vi "Qn10_X.vi"(11 "String":string) -> (3 "Qn":dbl[](array[numeric]))   [LabVIEW 2015]
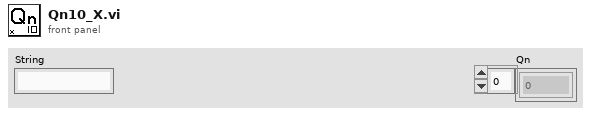
[diagram p1: front panel]
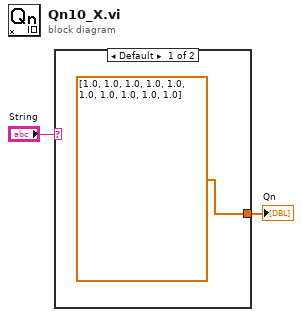
[diagram p0: block diagram]
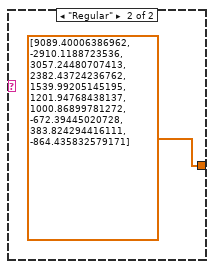
[diagram p2: hidden frame]
diagram:
  n1 = case shown="Default" "String" {
    tunnel: [dbl[] [1.0, 1.0, 1.0, 1.0, 1.0, 1.0, 1.0, 1.0, 1.0, 1.0] ("Qn") dbl[] [9089.40006386962, -2910.1188723536, 3057.24480707413, 2382.43724236762, 1539.99205145195, 1201.94768438137, 1000.86899781272, -672.39445020728, 383.824294416111, -864.435832579171] ("Qn")] -> w2
    frame Default {
    }
    frame "Regular" {
    }
  }
  "Qn" <- w2
